vi "match test.vi"   [LabVIEW 2021]
types:
  T1 = enum16{"Init", "Error", "Read", "Write", "Close"}
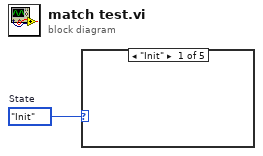
[diagram p0: block diagram]
diagram:
  w1 = T1."Init"  # State
  n1 = case shown="\"Init\"" w1 {
    frame "Init" {
    }
    frame "Error" {
    }
    frame "Read" {
    }
    frame "Write" {
    }
    frame "Close" {
    }
  }
